vi "Test_Convert_CameraAngle_to_Distance.vi"() -> ()   [LabVIEW 2019]
panel:
  out "Numeric":i32
  out "distances":dbl[](array[numeric])
  out "angles":dbl[](array[numeric])
  out "Test Plot":cluster{dbl[], dbl[]}(graph)
  out "a2":dbl
  out "d":dbl
  in  "StopValue":dbl=25.0
  in  "StartValue":dbl=-25.0
  in  "h1":dbl=20.56
  in  "h2":dbl=98.25
  in  "a1":dbl
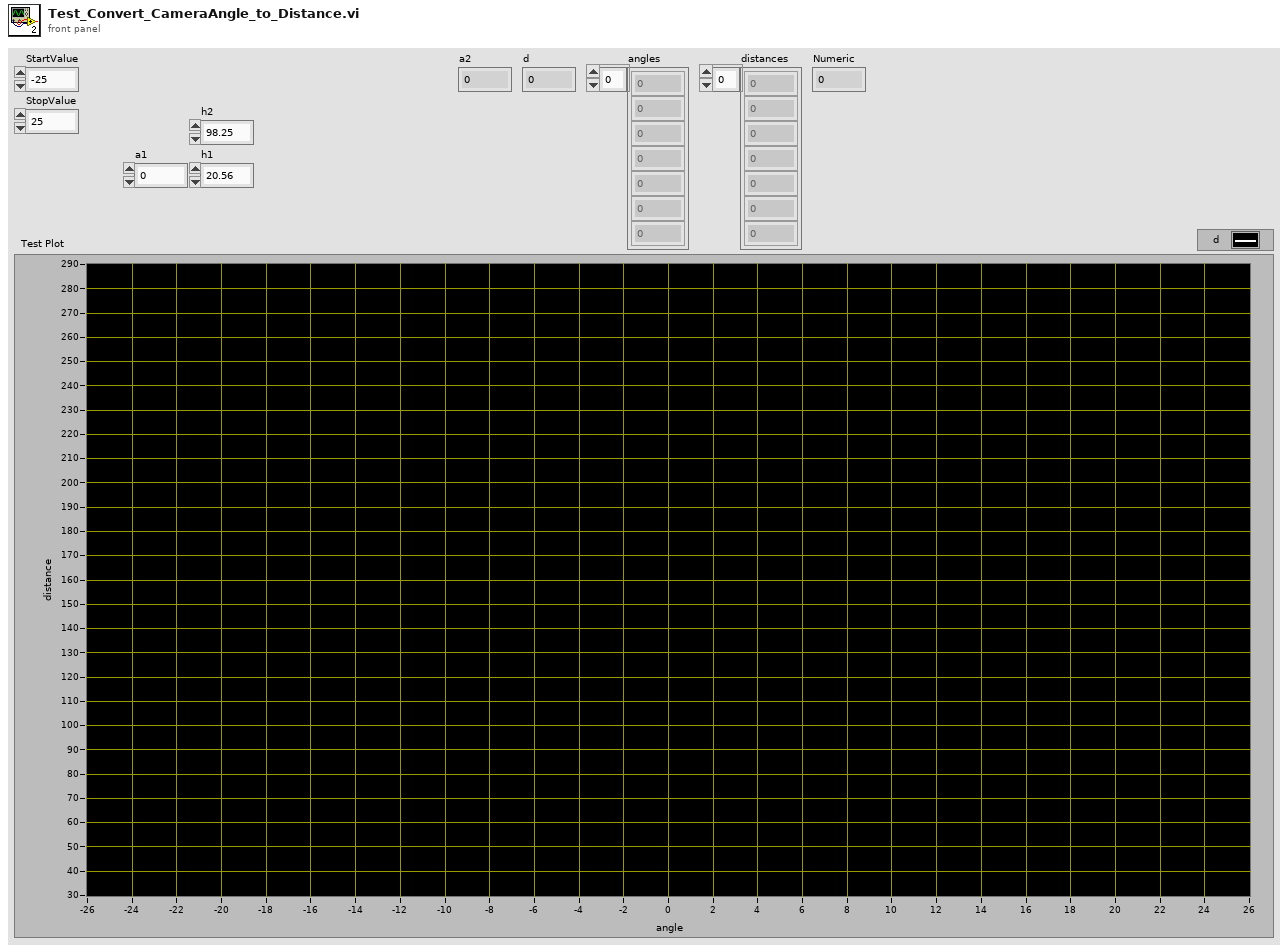
[diagram p1: front panel]
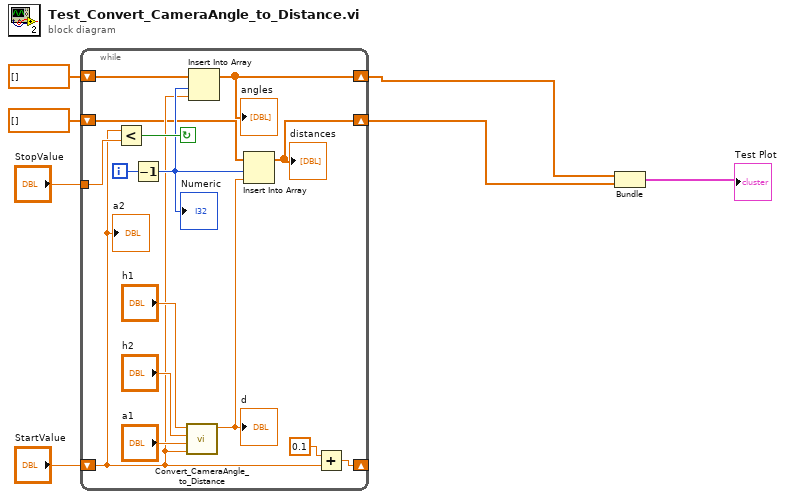
[diagram p0: block diagram]
diagram:
  n1 = while {
    shift-right: [w18] -> _
    shift-left: "StartValue" -> [w12]
    tunnel: "StopValue" -> [w17]
    shift-right: [w9] -> w3
    shift-left: dbl[] [] -> [w11]
    shift-right: [w8] -> w2
    shift-left: dbl[] [] -> [w10]
    i -> [w14]
    stop <- w16 continue-if-true
    n2 = Less?(x=w12, y=w17) -> (x < y?=w16:bool)
    n3 = Decrement(x=w14) -> (x-1=w13:i32)
    "Numeric" <- w13
    n4 = call "Convert_CameraAngle_to_Distance.vi"("a2"=w12, "a1"="a1", "h2"="h2", "h1"="h1") -> ("d"=w15:dbl)  [unwired: 7 in]
    "d" <- w15
    n5 = Insert Into Array(array=w11, index=w13, new element=w12) -> (w9:dbl[])
    "angles" <- w9
    n6 = Insert Into Array(array=w10, index=w13, new element=w15) -> (w8:dbl[])
    "distances" <- w8
    n7 = Add(x=0.1, y=w12) -> (x+y=w18:dbl)
    "a2" <- w12
  }
  n8 = Bundle(w3, w2) -> (→"Test Plot":cluster{dbl[], dbl[]})  [unwired: 1 in]
